vi "niRFUtil CONV 1 Ohm Voltage to dBm (real wfm).vi"(7 "Real Waveform (V)":T1 {"y" min=0 max=127 format="%.2f"; "dx" format="%^.2e"; "x0" format="%^.2e"}) -> (8 "Real Waveform (dBm)":T1 {"y" min=0 max=127 format="%.2f"; "dx" format="%^.2e"; "x0" format="%^.2e"})   [LabVIEW 2016, in "niRFUtil.lvlib"]
doc: "(c) Copyright 2006, National Instruments, Inc. This VI may not be duplicated, sold, or distributed without written consent from National Instruments."
uses:
  niRFUtil.lvlib
  Includes/niRFUtil INC Real Waveform.ctl
  Includes/niRFUtil INC Real Array.ctl
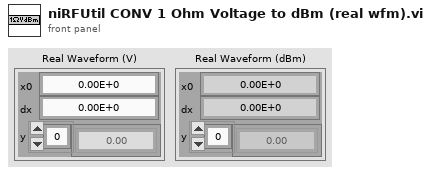
[diagram p1: front panel]
types:
  T1 = typedef "niRFUtil.lvlib/niRFUtil INC Real Waveform.ctl" = cluster{"x0":dbl, "dx":dbl, "y":T2}
  T2 = typedef "niRFUtil.lvlib/niRFUtil INC Real Array.ctl" = sgl[]
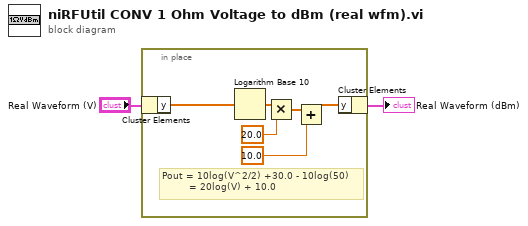
[diagram p0: block diagram]
diagram:
  n1 = in-place {
    # "Pout = 10log(V^2/2) +30.0 - 10log(50)\n         = 20log(V) + 10.0"
    n2 = in-place-cluster #1("Real Waveform (V)") -> ("y"=w4:T2)
    n3 = Logarithm Base 10(1:w4) -> (0:w8:T2)
    n4 = Multiply(x=w8, y=sgl 20.0) -> (x*y=w6:T2)
    n5 = Add(x=w6, y=sgl 10.0) -> (x+y=w3:T2)
    n6 = in-place-cluster #1("y"=w3) -> (→"Real Waveform (dBm)":T1)
  }
